vi "serialization tests.vi"() -> (0 "Pass":bool, 1 "Modules Equal":bool, 2 "Lines Equal Before Serial Test":bool, 3 "Lines Equal After Serial Test":bool, 4 "serialization error":errorcluster, 5 "Channels Equal":bool)   [LabVIEW 2014, in "io plugin tests.lvlib"]
doc: "Tests the 'To String' and 'From String' methods of the Module's configuration class and ensures they are compatible."
uses:
  io plugin tests.lvlib
  module/configuration/tag bus configurable plugin module configuration.lvclass
  module/configuration/tag bus configurable plugin module configuration.lvclass/tag bus configurable plugin module configuration.ctl
  <vilib>/NI/Tag Bus Module Framework/channel/TBM channel.lvclass
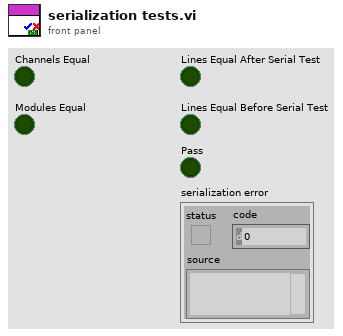
[diagram p1: front panel]
types:
  T1 = typedef "tag bus configurable plugin module configuration.lvclass/Line.ctl" = cluster{"channel":refnum<class "TBM channel.lvclass">}
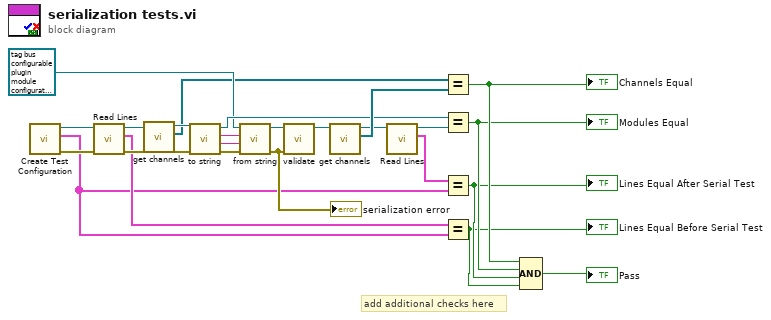
[diagram p0: block diagram]
diagram:
  # "add additional checks here"
  n1 = call "Create Test Configuration.vi"() -> ("error out"=w11:errorcluster, "Line Array"=w6:T1[], "Module Configuration"=w9:refnum<class "tag bus configurable plugin module configuration.lvclass">)  [unwired: 6 in, 3 out]
  n2 = call "Read Lines.vi"("error in (no error)"=w11, "tag bus configurable plugin module configuration in"=w9) -> ("error out"=w10:errorcluster, "Lines"=w7:T1[], "tag bus configurable plugin module configuration out"=w8:refnum<class "tag bus configurable plugin module configuration.lvclass">)  [unwired: 7 in]
  n3 = call-dynamic "get channels.vi"("module configuration in"=w8) -> ("channels"=w15:refnum<class "TBM channel.lvclass">[], "module configuration out"=w16:refnum<class "tag bus configurable plugin module configuration.lvclass">)  [unwired: 9 in]
  n4 = call-dynamic "to string.vi"("error in"=w10, "tag bus configurable plugin module configuration in"=w16) -> ("error out"=w25:errorcluster, "data"=w24:string, "version"=w23:string, "tag bus configurable plugin module configuration out"=w18:refnum<class "tag bus configurable plugin module configuration.lvclass">)  [unwired: 6 in]
  n5 = call-dynamic "from string.vi"("error in"=w25, "data"=w24, "version"=w23, "tag bus configurable plugin module configuration in"=refnum<class "tag bus configurable plugin module configuration.lvclass"> refnum ("tag bus configurable plugin module configuration")) -> ("error out"=w21:errorcluster, "tag bus configurable plugin module configuration out"=w22:refnum<class "tag bus configurable plugin module configuration.lvclass">)  [unwired: 6 in]
  "serialization error" <- w21
  n6 = call-dynamic "validate.vi"("error in"=w21, "tag bus configurable plugin module configuration in"=w22) -> ("tag bus configurable plugin module configuration out"=w20:refnum<class "tag bus configurable plugin module configuration.lvclass">)  [unwired: 8 in, 1 out]
  n7 = call-dynamic "get channels.vi"("module configuration in"=w20) -> ("channels"=w19:refnum<class "TBM channel.lvclass">[], "module configuration out"=w14:refnum<class "tag bus configurable plugin module configuration.lvclass">)  [unwired: 9 in]
  n8 = call "Read Lines.vi"("tag bus configurable plugin module configuration in"=w14) -> ("Lines"=w12:T1[], "tag bus configurable plugin module configuration out"=w13:refnum<class "tag bus configurable plugin module configuration.lvclass">)  [unwired: 8 in, 1 out]
  n9 = Equal?(x=w15, y=w19) -> (x = y?=w5:bool)
  "Channels Equal" <- w5
  n10 = Equal?(x=w18, y=w13) -> (x = y?=w4:bool)
  "Modules Equal" <- w4
  n11 = Equal?(x=w12, y=w6) -> (x = y?=w3:bool)
  "Lines Equal After Serial Test" <- w3
  n12 = Equal?(x=w7, y=w6) -> (x = y?=w2:bool)
  "Lines Equal Before Serial Test" <- w2
  n13 = Compound Arithmetic op=AND(w5, w4, w3, w2) -> (→"Pass":bool)
